vi "Spectrogram Plot.vi"(0 "FFT{I,Q}":dbl[][](array[numeric]) format="%.6f", 2 "Spectrogram parameters":T1 {"deltx" format="%.4f"; "delty" format="%.2f"; "y0" format="%.2f"}) -> (6 "Save data":bool caption="Boolean")   [LabVIEW 2022 SP3]
doc: "Vi takes the 2D array of numbers, of which each row corresponds to the magnitude of the FFT of the digitized doppler data"
panel:
  in  "Ring":u16(ring) items=["SAVE", "DON'T SAVE"]
  in  "Save Waveform":bool=TRUE caption="Boolean"
  out "Spectrogram":sgl[][](graph)
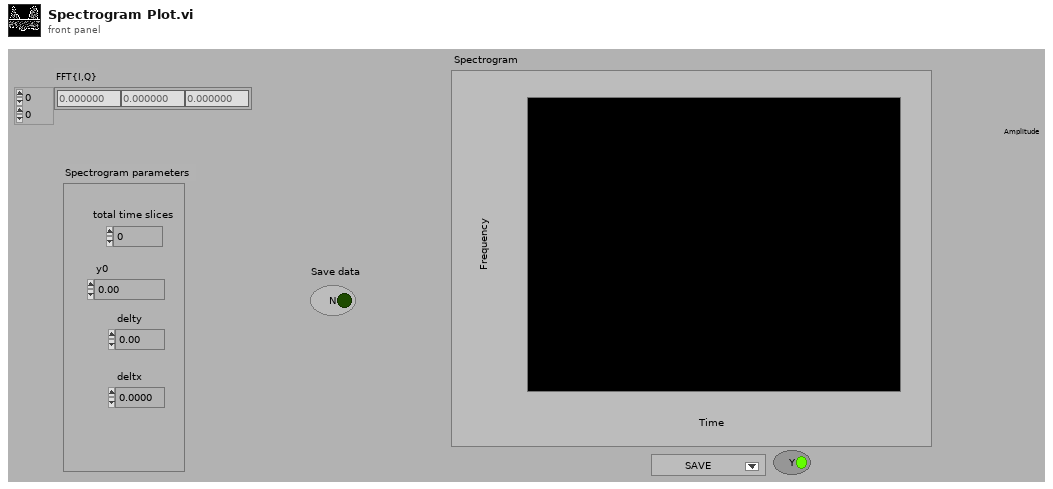
[diagram p1: front panel]
types:
  T1 = cluster{"total time slices":i32, "y0":dbl, "delty":dbl, "deltx":dbl}
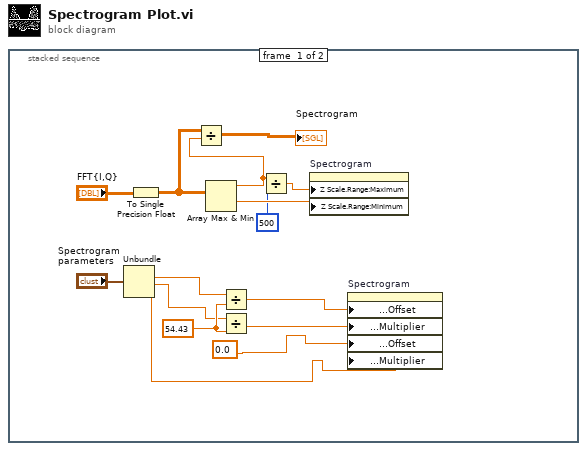
[diagram p0: block diagram]
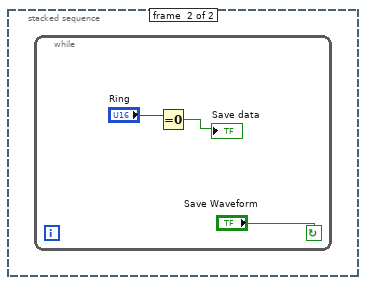
[diagram p2: hidden frame]
diagram:
  n1 = stacked-sequence {
    frame #0 {
      w13 = 54.43 ("frequency constant")
      n2 = Unbundle("Spectrogram parameters") -> ("y0"=w11:dbl, "delty"=w10:dbl, "deltx"=w5:dbl)  [unwired: 1 out]
      n3 = To Single Precision Float(number="FFT{I,Q}") -> (single precision float=w12:sgl[][])
      n4 = Array Max & Min(array=w12) -> (max value=w8:sgl, min value=w7:sgl)  [unwired: 2 out]
      n5 = Divide(x=w12, y=w8) -> (x/y=→"Spectrogram":sgl[][])
      n6 = Divide(x=w11, y=w13) -> (x/y=w4:dbl)
      n7 = Divide(x=w10, y=w13) -> (x/y=w3:dbl)
      n8 = Divide(x=w8, y=500) -> (x/y=w2:sgl)
      n9 = property on="Spectrogram" class="IntGraph (strict)"("Z Scale.Range:Maximum"=w2, "Z Scale.Range:Minimum"=w7) -> ()  [unwired: 2 in, 2 out]
      n10 = property on="Spectrogram" class="IntGraph (strict)"("Y Scale.Offset and Multiplier:Offset"=w4, "Y Scale.Offset and Multiplier:Multiplier"=w3, "X Scale.Offset and Multiplier:Offset"=0.0, "X Scale.Offset and Multiplier:Multiplier"=w5) -> ()  [unwired: 2 in, 2 out]
    }
    frame #1 {
      n11 = while {
        stop <- "Save Waveform" continue-if-true
        n12 = Equal To 0?(x="Ring") -> (x = 0?=→"Save data":bool)
      }
    }
  }
